vi "Camera Finder.vi"() -> (3 "IMAQ Interfaces":string[](array[string]))   [LabVIEW 2014]
uses:
  <vilib>/userdefined/High Color/IMAQdx.ctl
  <vilib>/vision/driver/NI_Vision_Acquisition_Software.lvlib
panel:
  out "Numeric":i32
  out "String":string
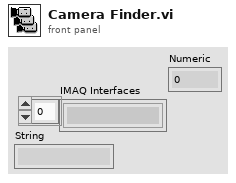
[diagram p1: front panel]
types:
  T1 = typedef "IMAQdx.ctl" = refnum<k21>
  T2 = typedef "IMAQ Image.ctl" = refnum<image>
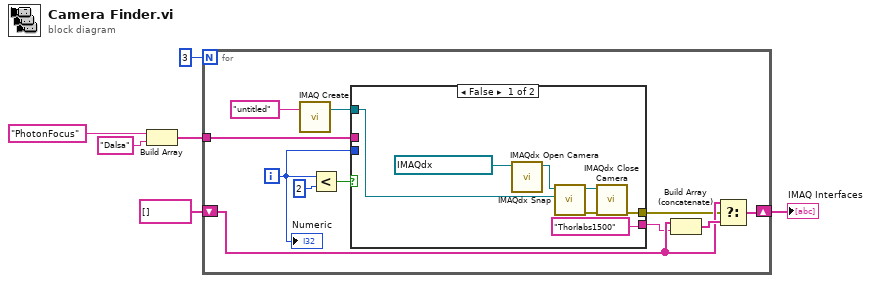
[diagram p0: block diagram]
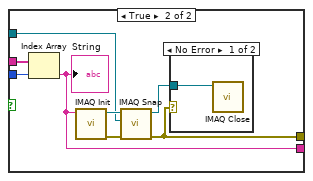
[diagram p2: hidden frame]
diagram:
  n1 = Build Array("PhotonFocus", "Dalsa") -> (w4:string[])
  n2 = for {
    N: 3 -> [_]
    tunnel: w4 -> [w9]
    shift-right: [w15] -> w5
    shift-left: string[] [] -> [w16]
    i -> [w8]
    n3 = call "IMAQ Create"("Image Name"="untitled") -> ("New Image"=w14:T2)  [unwired: 3 in, 2 out]
    n4 = Less?(x=w8, y=2) -> (x < y?=w11:bool)
    n5 = case shown="False" w11 {
      tunnel: w14 -> [w22 w29]
      tunnel: [w19 w28] -> w12
      tunnel: w9 -> [_ w27]
      tunnel: w8 -> [_ w26]
      tunnel: ["Thorlabs1500" w25] -> w7
      frame False {
        n6 = call <vilib>:"IMAQdx Open Camera.vi"("Session In"=T1 "Thorlabs1500") -> ("Session Out"=w23:T1)  [unwired: 9 in, 1 out]
        n7 = call <vilib>:"IMAQdx Snap.vi"("Image In"=w22, "Session In"=w23) -> ("error out"=w20:errorcluster, "Session Out"=w21:T1)  [unwired: 7 in, 1 out]
        n8 = call <vilib>:"IMAQdx Close Camera.vi"("error in"=w20, "Session In"=w21) -> ("error out"=w19:errorcluster)  [unwired: 9 in]
      }
      frame True {
        n9 = Index Array(array=w27, index=w26) -> (element=w25:string)
        "String" <- w25
        n10 = call <vilib>:"IMAQ Init.vi"("Interface Name"=w25) -> ("error out"=w30:errorcluster, "IMAQ Session Out"=w32:refnum<k11>)  [unwired: 9 in]
        n11 = call <vilib>:"IMAQ Snap.vi"("error in (no error)"=w30, "Image In"=w29, "IMAQ Session In"=w32) -> ("error out"=w28:errorcluster, "IMAQ Session Out"=w31:refnum<k11>)  [unwired: 6 in, 1 out]
        n12 = case shown="No Error" w28 {
          tunnel: w31 -> [w33 _]
          frame No Error {
            n13 = call <vilib>:"IMAQ Close.vi"("IMAQ Session In"=w33) -> ()  [unwired: 10 in, 1 out]
          }
          frame Error {
          }
        }
      }
    }
    n14 = Build Array (concatenate)(w16, w7) -> (w17:string[])
    n15 = Select(t=w16, s=w12, f=w17) -> (s? t:f=w15:string[])
    "Numeric" <- w8
  }
  "IMAQ Interfaces" <- w5
